vi "Write Update Water Level Msg.vi"(10 "更新水位消息":refnum<class "Update Water Level Msg.lvclass">, 11 "水位输入":refnum<class "Water Level.lvclass">) -> (3 "水位输出":refnum<class "Water Level.lvclass">)   [LabVIEW 2015, in "Water Level.lvlib" / "Water Level.lvclass"]
doc: "将更新水位消息（用于发送关于水深的更新）发送至调用方。调用方操作者在调用Launch Actor.vi之前设置该消息。"
uses:
  Water Level.lvclass
  Update Water Level Msg/Update Water Level Msg.lvclass
  Water Level.lvclass/Water Level.ctl
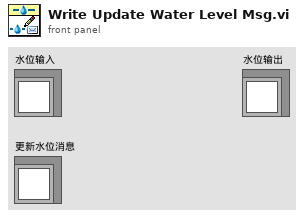
[diagram p1: front panel]
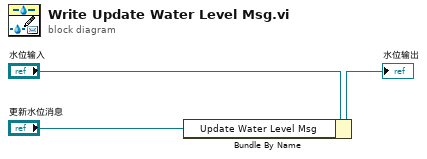
[diagram p0: block diagram]
diagram:
  n1 = Bundle By Name(cluster="水位输入", "Update Water Level Msg"="更新水位消息") -> (→"水位输出":refnum<class "Water Level.lvclass">)
